vi "Command Loop - Set HW Values.vi"(8 "error in":errorcluster, 10 "Data":string, 11 "Queue Refs in":T1) -> (0 "error out":errorcluster, 2 "Response":string, 3 "Queue Refs out":T1)   [LabVIEW 2025, in "Runtime Configuration Support Example Engine.lvlib"]
uses:
  Runtime Configuration Support Example Engine.lvlib
  Shared/Compiled.Settings.ctl
  <vilib>/NI VeriStand/Custom Device API/Custom Device Item Ref.ctl
  <vilib>/NI VeriStand/Custom Device API/Custom Device API.lvlib
  Shared/Runtime Configuration Support Example Shared.lvlib
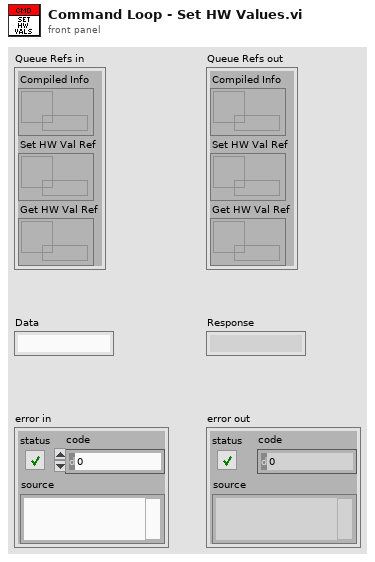
[diagram p1: front panel]
types:
  T1 = cluster{"Compiled Info":refnum<queue>, "Set HW Val Ref":refnum<queue>, "Get HW Val Ref":refnum<queue>}
  T2 = cluster{"SignalIDs":i32[], "Values":i32[], "Response Ref":refnum<queue>}
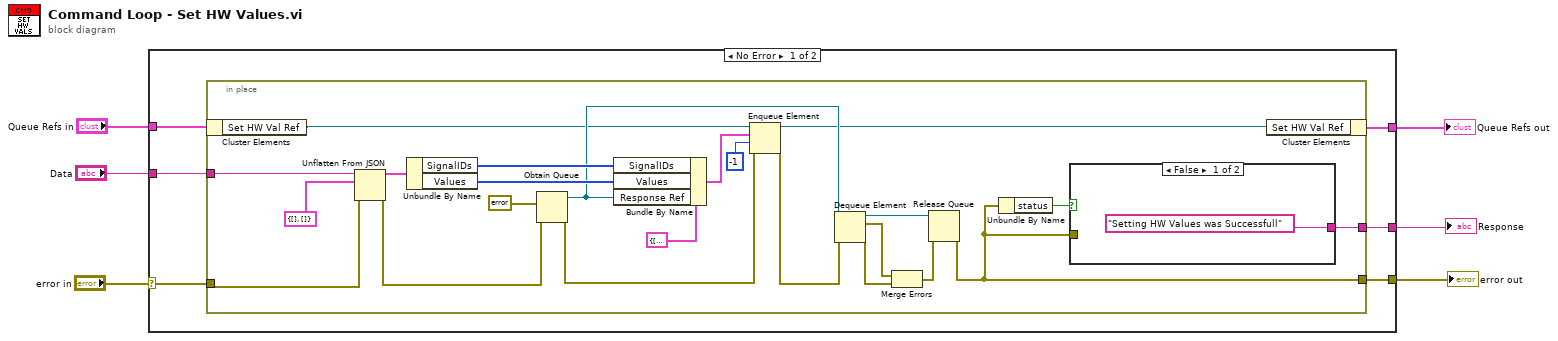
[diagram p0: block diagram]
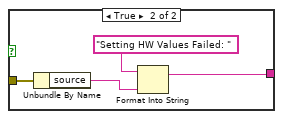
[diagram p2: hidden frame]
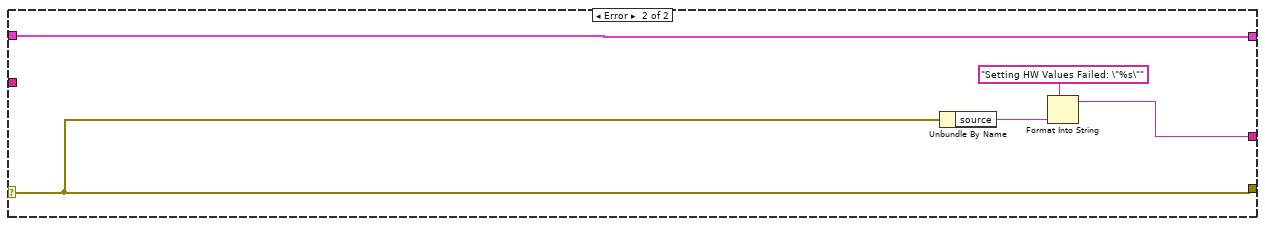
[diagram p3: hidden frame]
diagram:
  n1 = case shown="No Error" "error in" {
    selector: "error in" -> [w12 w45]
    tunnel: "Data" -> [w10 _]
    tunnel: "Queue Refs in" -> [w8 w41]
    tunnel: [w9 w42] -> w3
    tunnel: [w11 w45] -> w5
    tunnel: [w7 w41] -> w1
    frame No Error {
      n2 = in-place {
        in-place-border: w12 -> [w31]
        in-place-border: [w29] -> w11
        in-place-border: w10 -> [w20]
        in-place-border: [w17] -> w9
        n3 = in-place-cluster #1(w8) -> ("Set HW Val Ref"=w16:refnum<queue>)
        n4 = Unflatten From JSON(JSON string=w20, type and defaults=cluster{"SignalIDs":i32[], "Values":i32[]} {"SignalIDs"=[], "Values"=[]} ("element"), error in (no error)=w31) -> (value=w23:cluster{"SignalIDs":i32[], "Values":i32[]}, error out=w27:errorcluster)  [unwired: 4 in]
        n5 = Unbundle By Name(w23) -> ("SignalIDs"=w24:i32[], "Values"=w25:i32[])
        n6 = Obtain Queue(element data type=errorcluster {"status"=FALSE, "code"=0, "source"=""} ("error constant"), error in (no error)=w27) -> (queue out=w19:refnum<queue>, error out=w32:errorcluster)  [unwired: 3 in, 1 out]
        n7 = Bundle By Name(cluster=T2 {"SignalIDs"=[], "Values"=[], "Response Ref"=refnum}, "SignalIDs"=w24, "Values"=w25, "Response Ref"=w19) -> (w22:T2)
        n8 = Enqueue Element(queue=w16, element=w22, timeout in ms (-1)=-1, error in (no error)=w32) -> (queue out=w15:refnum<queue>, error out=w28:errorcluster)  [unwired: 1 out]
        n9 = Dequeue Element(queue=w19, error in (no error)=w28) -> (queue out=w13:refnum<queue>, element=w35:errorcluster, error out=w34:errorcluster)  [unwired: 1 in, 1 out]
        n10 = Merge Errors(w35, w34) -> (w30:errorcluster)
        n11 = Release Queue(queue=w13, error in (no error)=w30) -> (error out=w29:errorcluster)  [unwired: 1 in, 2 out]
        n12 = Unbundle By Name(w29) -> ("status"=w18:bool)
        n13 = case shown="False" w18 {
          tunnel: ["Setting HW Values was Successfull" ("format string") w38] -> w17
          tunnel: w29 -> [_ w40]
          frame False {
          }
          frame True {
            n14 = Unbundle By Name(w40) -> ("source"=w39:string)
            n15 = Format Into String(initial string="Setting HW Values Failed: " ("format string"), w39) -> (resulting string=w38:string)  [unwired: 2 in, 1 out]
          }
        }
        n16 = in-place-cluster #1("Set HW Val Ref"=w15) -> (w7:T1)
      }
    }
    frame Error {
      n17 = Unbundle By Name(w45) -> ("source"=w43:string)
      n18 = Format Into String(format string="Setting HW Values Failed: \"%s\"", w43) -> (resulting string=w42:string)  [unwired: 2 in, 1 out]
    }
  }
  "error out" <- w5
  "Response" <- w3
  "Queue Refs out" <- w1
